vi "Set Running.vi"(8 "error in (no error)":errorcluster, 10 "Running":bool, 11 "ArrayManager in":refnum<class "ArrayManager.lvclass">) -> (0 "error out":errorcluster, 3 "ArrayManager out":refnum<class "ArrayManager.lvclass">)   [LabVIEW 2020, in "OOPanel.lvlib" / "ArrayManager.lvclass"]
uses:
  ArrayManager.lvclass
  ArrayManager.lvclass/ArrayManager.ctl
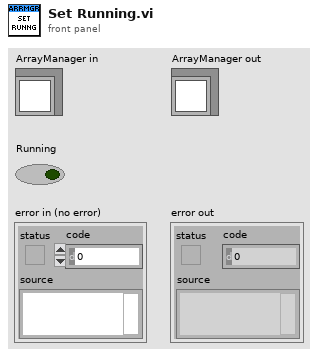
[diagram p1: front panel]
types:
  T1 = typedef "OOPanel.lvlib/ArrayManager.lvclass/State Ref.ctl" = cluster{"Running":bool, "Borders":bool, "Total Height":dbl, "Scroll Visible":bool, "Background":u32}
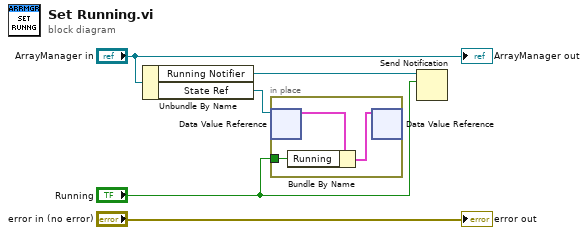
[diagram p0: block diagram]
diagram:
  n1 = Unbundle By Name("ArrayManager in") -> ("Running Notifier"=w2:refnum<notifier>, "State Ref"=w4:refnum<data-value>)
  n2 = in-place {
    in-place-border: "Running" -> [w6]
    n3 = in-place-dvr #1(w4) -> (w8:T1)  [unwired: 1 out]
    n4 = Bundle By Name(cluster=w8, "Running"=w6) -> (w7:T1)
    n5 = in-place-dvr #1(w7) -> ()  [unwired: 2 out]
  }
  n6 = Send Notification(notification="Running", notifier=w2) -> ()  [unwired: 1 in, 2 out]
  "error out" <- "error in (no error)"
  "ArrayManager out" <- "ArrayManager in"
